vi "two_button.vi"(7 "callee":refnum<vi>, 8 "error in (no error)":errorcluster, 10 "configuration":T2, 11 "v1 in":refnum<class "v1.lvclass">) -> (0 "error out":errorcluster, 2 "dialog_selection":T1, 3 "v1 out":refnum<class "v1.lvclass">)   [LabVIEW 2015, in "lv-dialog.lvlib" / "v1.lvlib" / "v1.lvclass"]
doc: "This approximates the functionality of the built-in two button dialog; the api has inputs for the message it displays and the text on each of the two buttons. On return it will indicate the interaction with the dialog (generally button_1, button_2 or panel_closed).\n\nThis IS implemented by the base api class using the built-in two button dialog."
uses:
  v1.lvclass
  _controls/selection.ctl
  v1.lvlib
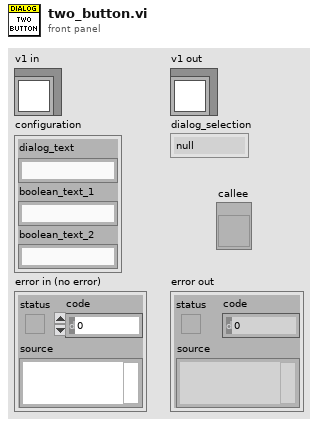
[diagram p1: front panel]
types:
  T1 = typedef "lv-dialog.lvlib/v1.lvlib/selection.ctl" = enum16{"null", "panel_closed", "button_1", "button_2", "button_3", "cancelled"}
  T2 = cluster{"dialog_text":string, "boolean_text_1":string, "boolean_text_2":string}
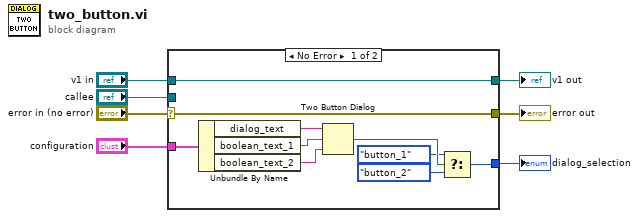
[diagram p0: block diagram]
diagram:
  n1 = case shown="No Error" "error in (no error)" {
    selector: "error in (no error)" -> [w16 w19]
    tunnel: [w16 w19] -> w6
    tunnel: [w17 w18] -> w4
    tunnel: "v1 in" -> [w17 w18]
    tunnel: "callee" -> [_ _]
    tunnel: "configuration" -> [w15 _]
    tunnel: [w8 _] -> w1
    frame No Error {
      n2 = Unbundle By Name(w15) -> ("dialog_text"=w14:string, "boolean_text_1"=w13:string, "boolean_text_2"=w12:string)
      n3 = Two Button Dialog(message=w14, 1:w12, 2:w13) -> (T button?=w11:bool)
      n4 = Select(t=selection."button_1" ("dialog_selection"), s=w11, f=selection."button_2" ("dialog_selection")) -> (s? t:f=w8:T1)
    }
    frame Error {
    }
  }
  "error out" <- w6
  "v1 out" <- w4
  "dialog_selection" <- w1
